vi "Arroyo TECSource Test.vi"() -> ()   [LabVIEW 2013]
panel:
  out "Num Terms":i16
  in  "Get constants":bool
  out "R0":dbl
  out "C3":dbl
  out "C2":dbl
  out "C1":dbl
  in  "TEC On":bool
  out "Current":dbl format="%.2g"
  out "Voltage":dbl format="%.2g"
  in  "SetTemp":bool
  in  "Setpoint":dbl=25.0 min=-99.0 max=250.0 step=0.01 format="%.2g"
  in  "Run":bool
  out "Temp":dbl format="%.2g"
  in  "COM Port":u16=4
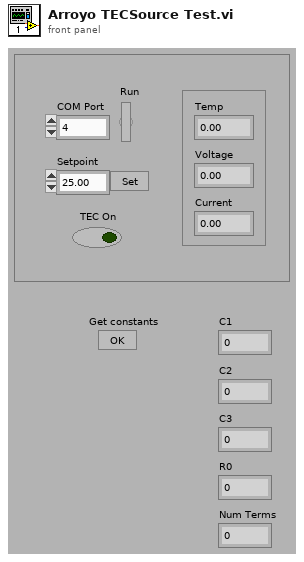
[diagram p1: front panel]
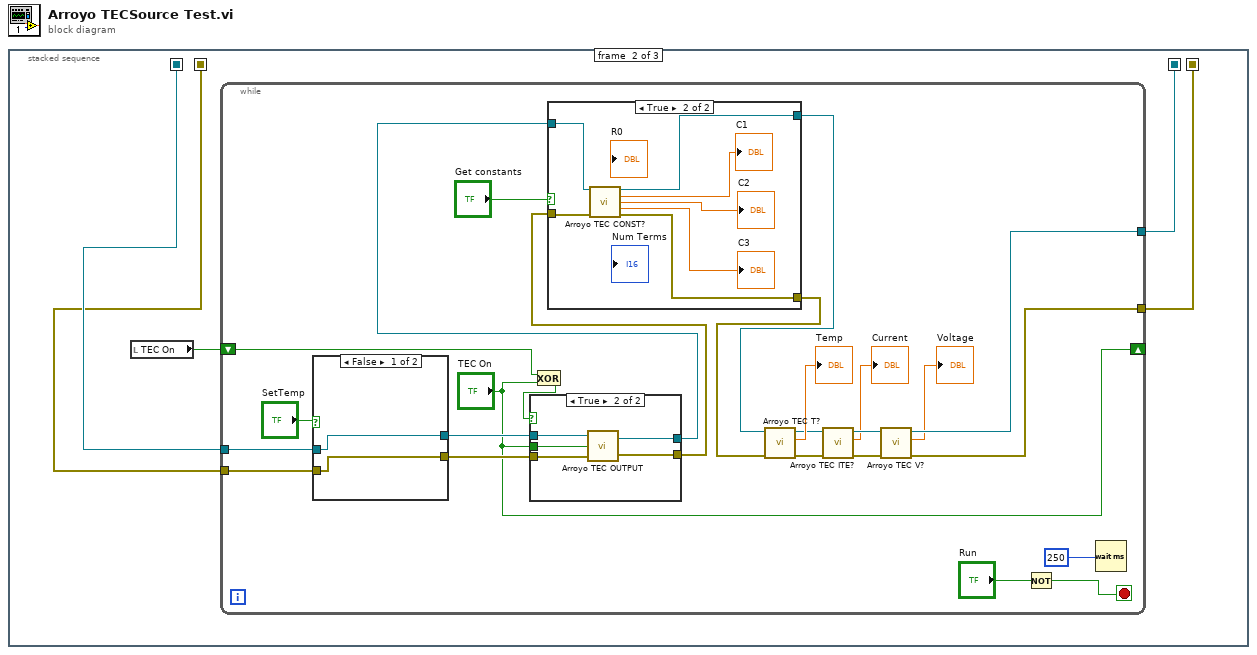
[diagram p0: block diagram]
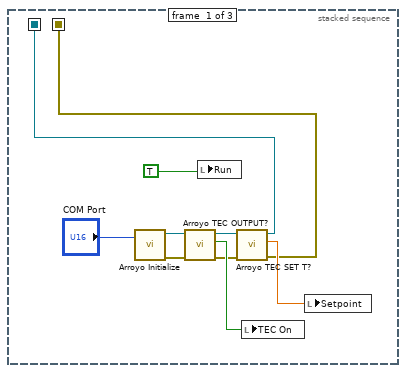
[diagram p2: hidden frame]
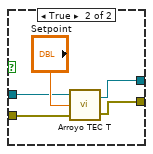
[diagram p5: hidden frame]
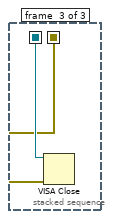
[diagram p6: hidden frame]
diagram:
  n1 = stacked-sequence {
    seq-local: [w5 _ _] -> [_ w12 _]
    seq-local: [w4 _ _] -> [_ w11 _]
    seq-local: [_ w15 _] -> [_ _ w65]
    seq-local: [_ w14 _] -> [_ _ w64]
    frame #0 {
      n2 = call "Arroyo Initialize.vi"("COM Port"="COM Port") -> ("dup VISA resource name"=w2:refnum<visa-resource-name>, "error out"=w3:errorcluster)  [unwired: 3 in]
      n3 = call "Arroyo TEC OUTPUT?.vi"("error in (no error)"=w3, "VISA resource name"=w2) -> ("error out"=w8:errorcluster, "TEC Output"=w9:bool, "dup VISA resource name"=w7:refnum<visa-resource-name>)  [unwired: 3 in]
      n4 = local write "Run"(TRUE) -> ()
      n5 = call "Arroyo TEC SET T?.vi"("error in (no error)"=w8, "VISA resource name"=w7) -> ("error out"=w4:errorcluster, "TEC Temperature Setpoint"=w10:dbl, "dup VISA resource name"=w5:refnum<visa-resource-name>)  [unwired: 3 in]
      n6 = local write "TEC On"(w9) -> ()
      n7 = local write "Setpoint"(w10) -> ()
    }
    frame #1 {
      n8 = local read "TEC On"() -> (w13:bool)
      n9 = while {
        tunnel: [w28] -> w14
        tunnel: [w32] -> w15
        shift-right: ["TEC On"] -> _
        shift-left: w13 -> [w27]
        tunnel: w12 -> [w22]
        tunnel: w11 -> [w21]
        stop <- w36 stop-if-true
        n10 = case shown="False" "SetTemp" {
          tunnel: [w57 w62] -> w25
          tunnel: [w58 w61] -> w24
          tunnel: w22 -> [w58 w60]
          tunnel: w21 -> [w57 w59]
          frame False {
          }
          frame True {
            n11 = call "Arroyo TEC T.vi"("error in (no error)"=w59, "TEC Temperature Setpoint"="Setpoint", "VISA resource name"=w60) -> ("error out"=w62:errorcluster, "dup VISA resource name"=w61:refnum<visa-resource-name>)
          }
        }
        n12 = Exclusive Or(1:"TEC On", 2:w27) -> (0:w26:bool)
        n13 = case shown="True" w26 {
          tunnel: "TEC On" -> [_ w56]
          tunnel: w25 -> [w50 w55]
          tunnel: w24 -> [w51 w54]
          tunnel: [w51 w53] -> w19
          tunnel: [w50 w52] -> w18
          frame False {
          }
          frame True {
            n14 = call "Arroyo TEC OUTPUT.vi"("error in (no error)"=w55, "TEC Output Enable"=w56, "VISA resource name"=w54) -> ("error out"=w52:errorcluster, "dup VISA resource name"=w53:refnum<visa-resource-name>)
          }
        }
        n15 = case shown="True" "Get constants" {
          tunnel: w19 -> [w42 w49]
          tunnel: w18 -> [w41 w48]
          tunnel: [w41 w46] -> w17
          tunnel: [w42 w47] -> w16
          frame False {
          }
          frame True {
            n16 = call "Arroyo TEC CONST?.vi"("VISA resource name"=w49, "error in (no error)"=w48) -> ("dup VISA resource name"=w47:refnum<visa-resource-name>, "C1"=→"C1":dbl, "C2"=→"C2":dbl, "C3"=→"C3":dbl, "error out"=w46:errorcluster)  [unwired: 7 in, 2 out]
          }
        }
        n17 = call "Arroyo TEC T?.vi"("error in (no error)"=w17, "VISA resource name"=w16) -> ("error out"=w33:errorcluster, "TEC Temperature"=→"Temp":dbl, "dup VISA resource name"=w39:refnum<visa-resource-name>)  [unwired: 3 in]
        n18 = call "Arroyo TEC ITE?.vi"("error in (no error)"=w33, "VISA resource name"=w39) -> ("error out"=w31:errorcluster, "TEC Current"=→"Current":dbl, "dup VISA resource name"=w34:refnum<visa-resource-name>)  [unwired: 3 in]
        n19 = call "Arroyo TEC V?.vi"("error in (no error)"=w31, "VISA resource name"=w34) -> ("error out"=w28:errorcluster, "TEC Voltage"=→"Voltage":dbl, "dup VISA resource name"=w32:refnum<visa-resource-name>)  [unwired: 3 in]
        n20 = Not(x="Run") -> (.not. x?=w36:bool)
        n21 = Wait (ms)(milliseconds to wait=250) -> ()  [unwired: 1 out]
      }
    }
    frame #2 {
      n22 = VISA Close(VISA resource name=w65, error in (no error)=w64) -> ()  [unwired: 1 out]
    }
  }
